vi "PH_Timing.Set 0-5HzGater.vi"(0 "i ref in":refnum<vi>, 5 "error in (no error)":errorcluster) -> (14 "i ref out":refnum<vi>, 19 "error out":errorcluster)   [LabVIEW 2014, in "PH_Timing.lvlib"]
doc: "This VI sets the 0,5Hz-Gater configuration."
uses:
  PH_Timing.lvlib
  CS_DigitalIO/BNC555/BNC555.lvlib
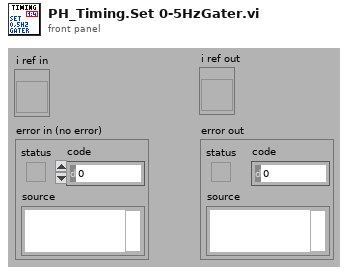
[diagram p1: front panel]
types:
  T1 = enum16{"Normal", "Single", "Burst", "Duty Cycle"}
  T2 = typedef "PH_Timing.lvlib/PH_Timing.i attribute.ctl" = cluster{"Sequencer":cluster{"linked?":bool, "Proc State":string, "Ref State":refnum<vi>}, "Gate Generator":cluster{"GD":cluster{"Device Status":T3, "linked?":bool}, "Settings":T4, "GUI Ref":refnum<vi>}, "Interlock Bypass":cluster{"Instancename":string, "Switch linked?":bool, "Device Status":T3, "Ref Status":refnum<vi>}, "Roughtuner":cluster{"Settings":T5, "GUI Ref":refnum<vi>, "GD":cluster{"Device Status":T3, "linked?":bool}}, "0,5Hz Gater":cluster{"Settings":T6, "GUI Ref":refnum<vi>, "GD":cluster{"Device Status":T3, "linked?":bool}}, "Slow Trigger":cluster{"Settings":T7, "GUI Ref":refnum<vi>, "Service ID Delay":i32, "Service ID Ext Trig":i32, "Wanted Settings":T7}, "Timing Mode":cluster{"Mode":T8, "GUI Ref":refnum<vi>, "Service ID T2":i32, "Service ID Mode":i32, "Wanted Mode":T8}, "ns Generator":cluster{"Settings":T9, "ns Generator Settings":refnum<vi>, "GD":cluster{"Device Status":T3, "linked?":bool}}, "Phase FEs":cluster{"Settings":T12, "GUI Ref":refnum<vi>, "Service ID Phase":i32, "Wanted Settings":T12}, "GD GUI Refs":refnum<vi>[], "Heads":T13[], "GUI Ref Delete":refnum<vi>}
  T3 = typedef "PH_StatusHandler.lvlib/PH_StatusHandler.Status.ctl" = i16
  T4 = typedef "PH_Timing.lvlib/PH_Timing.GateGen.ctl" = cluster{"Instance":string, "Channel Gate":i32, "Channel T2":i32, "Width Gate":dbl, "Width T2":dbl, "Delay Gate":dbl, "Delay T2":dbl, "Gate activ":bool, "T2 activ":bool, "System Mode":enum16{"Normal", "Single", "Burst", "Duty Cycle"}}
  T5 = typedef "PH_Timing.lvlib/PH_Timing.Roughtuner.ctl" = cluster{"Instance":string, "Phase PHELIX / UNILAC":cluster{"Channel":u16, "relative to":u16, "Delay [ms]":dbl}, "Pulse Length":cluster{"Channel":u16, "relative to":u16, "Delay [ms]":dbl}, "Trigger":cluster{"externally?":bool, "Rate [Hz]":dbl}}
  T6 = typedef "PH_Timing.lvlib/PH_Timing.0.5HzGater.ctl" = cluster{"Instance":string, "Channel ns FE Delay":i32, "Channel 0.5Hz":i32, "Width ns FE Delay":dbl, "Width 0.5Hz":dbl, "Delay ns FE Delay":dbl, "Delay 0.5Hz":dbl, "ns FE Delay active":bool, "0.5Hz activ":bool, "ns FE Delay inverted":bool, "0.5Hz inverted":bool}
  T7 = typedef "PH_Timing.lvlib/PH_Timing.Slow Trigger Settings.ctl" = cluster{"Delay":dbl, "externally triggered?":bool}
  T8 = typedef "PH_Timing.lvlib/PH_Timing.Timing Mode.ctl" = cluster{"T2":i16, "Modeselector":enum32{"10 Hz", "0.5 Hz", "Shot"}}
  T9 = typedef "PH_Timing.lvlib/PH_Timing.ns Generator.ctl" = cluster{"Instance":string, "Phase fs / ns FE":cluster{"Channel":T10, "Settings":T11}}
  T10 = typedef "Stanford Research DG645 - Driver.lvlib/Channel.ctl" = i32
  T11 = typedef "PH_SRDG645.lvlib/PH_SRDG645.Channel Settings.ctl" = cluster{"Delay [s]":dbl, "relative to":i32}
  T12 = typedef "PH_Timing.lvlib/PH_Timing.Phase FEs.ctl" = cluster{"Phase":dbl}
  T13 = typedef "PH_Timing.lvlib/PH_Timing.PU Data.ctl" = cluster{"linked?":bool, "Data":T14, "GD":cluster{"Device Status":T3, "linked?":bool}, "GUI Ref":refnum<vi>, "PU":T15}
  T14 = typedef "PH_Timing.lvlib/PH_Timing.PU Info.ctl" = cluster{"Act CH?":bool, "GD":string, "CH":i32, "Delay":dbl, "active":bool, "in Use?":bool}
  T15 = typedef "PH_PP_Common.lvlib/PH_PP_Common.PUs.ctl" = enum16{"no Info", "PA-19mm-1", "PA-19mm-2", "PA-45mm-PILC", "PA-45mm-MAIN", "MA-PU-1", "MA-PU-2", "MA-PU-3", "MA-PU-4", "MA-PU-5", "MA-PU-6", "MA-FR", "MA-PILC", "PA-45mm-DP"}
  T16 = enum16{"Normal", "Single", "Burst", "Divide by N"}
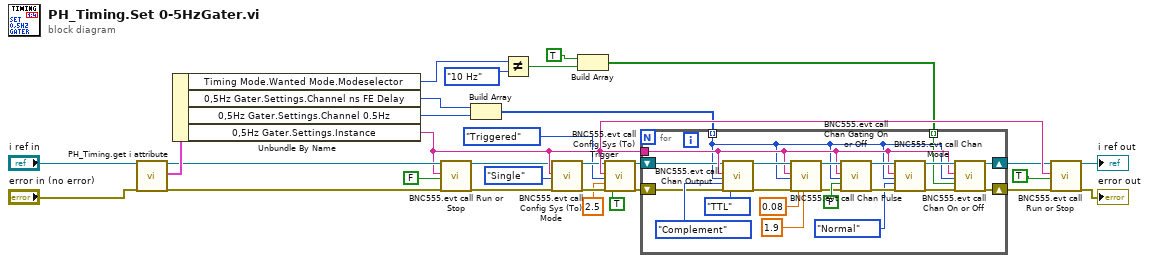
[diagram p0: block diagram]
diagram:
  n1 = call "PH_Timing.get i attribute.vi"("i ref in"="i ref in", "error in (no error)"="error in (no error)") -> ("i ref out"=w26:refnum<vi>, "i attribute"=w28:T2, "error out"=w27:errorcluster)  [unwired: 15 in]
  n2 = Unbundle By Name(w28) -> ("Timing Mode.Wanted Mode.Modeselector"=w4:enum32{"10 Hz", "0.5 Hz", "Shot"}, "0,5Hz Gater.Settings.Channel ns FE Delay"=w21:i32, "0,5Hz Gater.Settings.Channel 0.5Hz"=w22:i32, "0,5Hz Gater.Settings.Instance"=w23:string)
  n3 = call "BNC555.evt call Run or Stop.vi"("i ref in"=w26, "Generator Instance"=w23, "Start\\Stop"=FALSE ("Start\\Stop"), "error in (no error)"=w27) -> ("i ref out"=w9:refnum<vi>, "error out"=w8:errorcluster)  [unwired: 14 in]
  n4 = Build Array(w21, w22) -> (w20:i32[])
  n5 = Not Equal?(x=w4, y=enum32{"10 Hz", "0.5 Hz", "Shot"}."10 Hz" ("Timing Mode.Wanted Mode.Modeselector")) -> (x != y?=w1:bool)
  n6 = call "BNC555.evt call Config Sys (To) Mode.vi"("i ref in"=w9, "Generator Instance"=w23, "Mode"=T1."Single", "error in (no error)"=w8) -> ("i ref out"=w19:refnum<vi>, "error out"=w18:errorcluster)  [unwired: 14 in]
  n7 = Build Array(TRUE, w1) -> (w6:bool[])
  n8 = call "BNC555.evt call Config Sys (To) Trigger.vi"("i ref in"=w19, "Generator Instance"=w23, "Mode"=enum16{"Disabled", "Triggered", "Gated"}."Triggered", "Trigger Level (2.5V)"=2.5 ("Trigger Level [V] (0.5)"), "error in (no error)"=w18, "Trigger Edge (T:Rising)"=TRUE) -> ("i ref out"=w17:refnum<vi>, "error out"=w16:errorcluster)  [unwired: 12 in]
  n9 = for {
    shift-right: [w45] -> w12
    shift-left: w17 -> [w37]
    shift-right: [w47] -> w11
    shift-left: w16 -> [w36]
    tunnel: w23 -> [w39]
    tunnel: w20 -> [w35] mode=indexing
    tunnel: w6 -> [w31] mode=indexing
    n10 = call "BNC555.evt call Chan Output.vi"("i ref in"=w37, "Generator Instance"=w39, "Channel"=w35, "Polarity (Normal)"=enum16{"Normal", "Complement", "Inverted"}."Complement", "error in (no error)"=w36, "Level (TTL)"=enum16{"TTL", "Adjustable", "35 Volt"}."TTL") -> ("i ref out"=w41:refnum<vi>, "error out"=w40:errorcluster)  [unwired: 12 in]
    n11 = call "BNC555.evt call Chan Pulse.vi"("i ref in"=w41, "Generator Instance"=w39, "Channel"=w35, "error in (no error)"=w40, "Delay"=0.08, "Width"=1.9) -> ("i ref out"=w44:refnum<vi>, "error out"=w43:errorcluster)  [unwired: 12 in]
    n12 = call "BNC555.evt call Chan Gating On or Off.vi"("i ref in"=w44, "Generator Instance"=w39, "Channel"=w35, "Gating State"=FALSE ("Gate enabled (false)"), "error in (no error)"=w43) -> ("i ref out"=w49:refnum<vi>, "error out"=w50:errorcluster)  [unwired: 13 in]
    n13 = call "BNC555.evt call Chan Mode.vi"("i ref in"=w49, "Generator Instance"=w39, "Channel"=w35, "Mode"=T16."Normal" ("Mode (0:Normal)"), "error in (no error)"=w50) -> ("i ref out"=w46:refnum<vi>, "error out"=w48:errorcluster)  [unwired: 13 in]
    n14 = call "BNC555.evt call Chan On or Off.vi"("i ref in"=w46, "Generator Instance"=w39, "Channel"=w35, "State"=w31, "error in (no error)"=w48) -> ("i ref out"=w45:refnum<vi>, "error out"=w47:errorcluster)  [unwired: 13 in]
  }
  n15 = call "BNC555.evt call Run or Stop.vi"("i ref in"=w12, "Generator Instance"=w23, "Start\\Stop"=TRUE, "error in (no error)"=w11) -> ("i ref out"=→"i ref out":refnum<vi>, "error out"=→"error out":errorcluster)  [unwired: 14 in]
